vi "Get Stream Support Info.vi"(8 "error in (no error)":errorcluster, 9 "Device Number":string, 11 "VISA resource name":refnum<visa-resource-name>) -> (0 "error out":errorcluster, 1 "Number of Buffers":i32, 2 "Number of Streams":i32, 3 "VISA resource name out":refnum<visa-resource-name>)   [LabVIEW 2018, in "Zaber A Series.lvlib"]
doc: "Returns information about the device's support for streaming commands, namely the number of simultaneous streams supported (or 0 if streaming is not available), and the number of buffers available for saved streams.\n\nThis VI requires that the Initialize VI has been called with the same serial port."
uses:
  Zaber A Series.lvlib
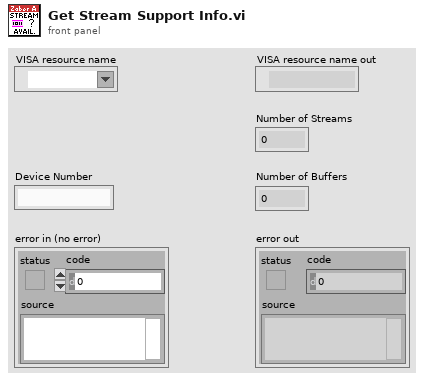
[diagram p1: front panel]
types:
  T1 = cluster{"Device":string, "Axis":string, "Reply Flag":string, "Status":string, "Warning Flags":string, "Data":string}[]
  T2 = cluster{"Device":string, "Axis":string, "Reply Flag":string, "Status":string, "Warning Flags":string, "Data":string}
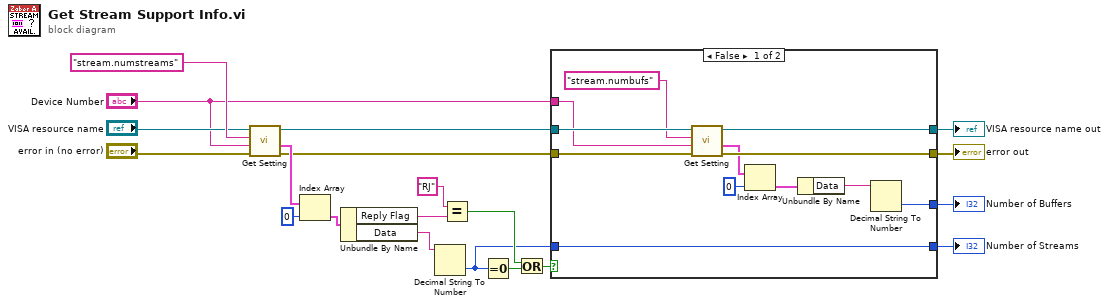
[diagram p0: block diagram]
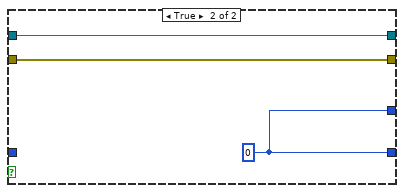
[diagram p2: hidden frame]
diagram:
  n1 = call "Get Setting.vi"("error in (no error)"="error in (no error)", "Device and Axis"="Device Number", "Setting"="stream.numstreams", "VISA resource name"="VISA resource name") -> ("error out"=w6:errorcluster, "Response Bundle Array"=w19:T1, "VISA resource name out"=w8:refnum<visa-resource-name>)  [unwired: 2 in, 3 out]
  n2 = Index Array(array=w19, index=0) -> (element=w17:T2)
  n3 = Unbundle By Name(w17) -> ("Reply Flag"=w2:string, "Data"=w1:string)
  n4 = Decimal String To Number(string=w1) -> (number=w10:i32)  [unwired: 2 in, 1 out]
  n5 = Equal?(x="RJ", y=w2) -> (x = y?=w14:bool)
  n6 = Equal To 0?(x=w10) -> (x = 0?=w15:bool)
  n7 = Or(x=w14, y=w15) -> (x .or. y?=w11:bool)
  n8 = case shown="False" w11 {
    tunnel: w10 -> [w32 _]
    tunnel: [w32 w33] -> w9
    tunnel: w8 -> [w31 w35]
    tunnel: [w29 w35] -> w7
    tunnel: w6 -> [w30 w34]
    tunnel: [w28 w34] -> w5
    tunnel: "Device Number" -> [w27 _]
    tunnel: [w21 w33] -> w3
    frame False {
      n9 = call "Get Setting.vi"("error in (no error)"=w30, "Device and Axis"=w27, "Setting"="stream.numbufs", "VISA resource name"=w31) -> ("error out"=w28:errorcluster, "Response Bundle Array"=w22:T1, "VISA resource name out"=w29:refnum<visa-resource-name>)  [unwired: 2 in, 3 out]
      n10 = Index Array(array=w22, index=0) -> (element=w24:T2)
      n11 = Unbundle By Name(w24) -> ("Data"=w25:string)
      n12 = Decimal String To Number(string=w25) -> (number=w21:i32)  [unwired: 2 in, 1 out]
    }
    frame True {
      w33 = 0
    }
  }
  "VISA resource name out" <- w7
  "error out" <- w5
  "Number of Streams" <- w9
  "Number of Buffers" <- w3
